vi "SMU-VSU name converter.vi"(1 "unit to configure":u32(slide) max=7 scale=0.0..7.0) -> (0 "SMU/VSU to be configured":string)   [LabVIEW 2016]
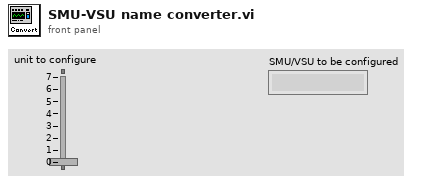
[diagram p1: front panel]
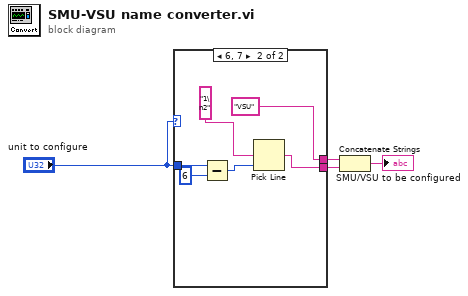
[diagram p0: block diagram]
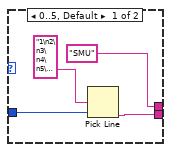
[diagram p2: hidden frame]
diagram:
  n1 = case shown="6, 7" "unit to configure" {
    tunnel: "unit to configure" -> [w7 w11]
    tunnel: ["SMU" "VSU"] -> w4
    tunnel: [w5 w12] -> w3
    frame 0..5, Default {
      n2 = Pick Line(multi-line string="1\n2\n3\n4\n5\n6", line index=w7) -> (output string=w5:string)  [unwired: 1 in]
    }
    frame 6, 7 {
      n3 = Subtract(x=w11, y=u32 6) -> (x-y=w9:u32)
      n4 = Pick Line(multi-line string="1\n2", line index=w9) -> (output string=w12:string)  [unwired: 1 in]
    }
  }
  n5 = Concatenate Strings(w4, w3) -> (→"SMU/VSU to be configured":string)
